vi "dfd_Bssl Lowpass S Poles and Zeros.vi"(2 "low cutoff freq: wl":dbl=0.125 format="%.3f", 3 "order":i32=2) -> (0 "zeros":T1[](array[typedef]), 1 "poles":T1[](array[typedef]))   [LabVIEW 2017, in "NI_DigFilter_Design.lvlib"]
uses:
  <vilib>/addons/Digital Filter Design/NI_DigFilter_Design.lvlib
  <vilib>/addons/Digital Filter Design/_Objects.llb/DFD Pole-Zero.ctl
  <vilib>/addons/Digital Filter Design/NI_DigFilterLicensed.lvlib
panel:
  in  "zp cluster":T1={"value"=0.0+0.0i, "z attr"={"real"=FALSE, "lp"=FALSE, "uc"=FALSE}, "order"=1}
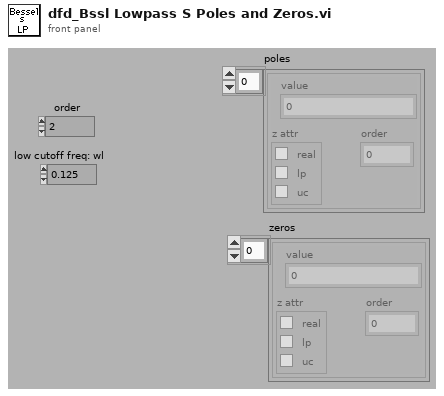
[diagram p1: front panel]
types:
  T1 = typedef "NI_DigFilterLicensed.lvlib/DFD Pole-Zero.ctl" = cluster{"value":cdb, "z attr":cluster{"real":bool, "lp":bool, "uc":bool}, "order":i32}
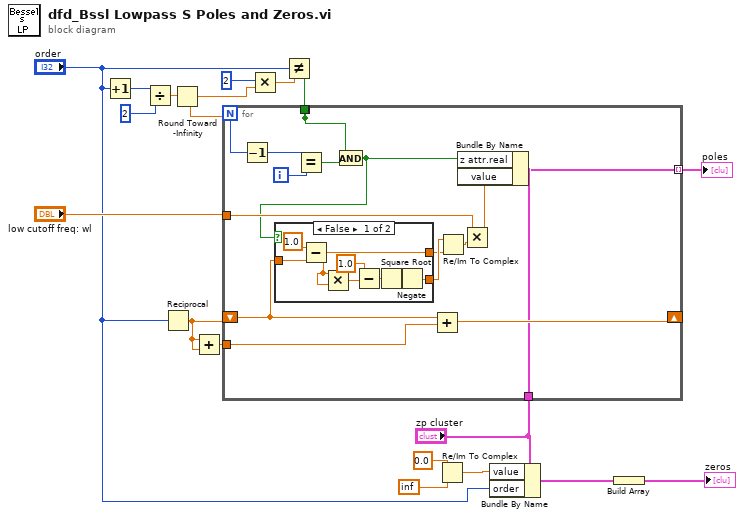
[diagram p0: block diagram]
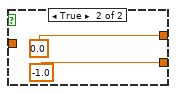
[diagram p2: hidden frame]
diagram:
  n1 = Increment(x="order") -> (x+1=w18:i32)
  n2 = Divide(x=w18, y=2) -> (x/y=w16:dbl)
  n3 = Reciprocal(x="order") -> (1/x=w3:dbl)
  n4 = Round Toward -Infinity(1:w16) -> (0:w11:dbl)
  n5 = Add(x=w3, y=w3) -> (x+y=w2:dbl)
  n6 = Multiply(x=2, y=w11) -> (x*y=w13:dbl)
  n7 = Not Equal?(x="order", y=w13) -> (x != y?=w12:bool)
  n8 = for {
    N: w11 -> [w29]
    shift-right: [w34] -> _
    shift-left: w3 -> [w20]
    tunnel: "low cutoff freq: wl" -> [w32]
    tunnel: "zp cluster" -> [w27]
    tunnel: [w25] -> _ mode=indexing
    tunnel: [w26] -> w15 mode=indexing
    tunnel: w12 -> [w25]
    tunnel: w2 -> [w19]
    i -> [w31]
    n9 = Decrement(x=w29) -> (x-1=w30:i32)
    n10 = Equal?(x=w30, y=w31) -> (x = y?=w28:bool)
    n11 = And(x=w25, y=w28) -> (x .and. y?=w21:bool)
    n12 = case shown="False" w21 {
      tunnel: w20 -> [w41 _]
      tunnel: [w35 -1.0] -> w23
      tunnel: [w38 0.0] -> w22
      frame False {
        n13 = Subtract(x=1.0, y=w41) -> (x-y=w38:dbl)
        n14 = Multiply(x=w38, y=w38) -> (x*y=w39:dbl)
        n15 = Subtract(x=1.0, y=w39) -> (x-y=w36:dbl)
        n16 = Square Root(x=w36) -> (sqrt(x)=w37:dbl)
        n17 = Negate(x=w37) -> (-x=w35:dbl)
      }
      frame True {
      }
    }
    n18 = Add(x=w20, y=w19) -> (x+y=w34:dbl)
    n19 = Re/Im To Complex(1:w22, 2:w23) -> (0:w33:cdb)
    n20 = Multiply(x=w32, y=w33) -> (x*y=w24:cdb)
    n21 = Bundle By Name(cluster=w27, "z attr.real"=w21, "value"=w24) -> (w26:T1)
  }
  "poles" <- w15
  n22 = Re/Im To Complex(1:inf, 2:0.0) -> (0:w6:cdb)
  n23 = Bundle By Name(cluster="zp cluster", "value"=w6, "order"="order") -> (w10:T1)
  n24 = Build Array(w10) -> (→"zeros":T1[])
